vi "SATPdll.vi"(8 "error in (no error)":errorcluster, 11 "SAT Inputs":cluster{"p":dbl, "z":dbl[], "kph":u16}={"p"=0.0, "z"=[0.0, 0.0, 0.0, 0.0, 0.0, 0.0, 0.0, 0.0, 0.0, 0.0, 0.0, 0.0, 0.0, 0.0, 0.0, 0.0, 0.0, 0.0, 0.0, 0.0], "kph"=4} {"kph" items=["1 = input x is liquid composition"=1, "2 = input x is vapor composition"=2, "3 = input x is liquid composition (freezing point)"=3, "4 = input x is vapor composition (sublimation point)"=4]}) -> (0 "error out":errorcluster, 3 "SAT Outputs":T1={"D"=nan, "e"=nan, "h"=nan, "p"=nan, "s"=nan, "t"=nan, "q"=nan, "Dl"=nan, "Dv"=nan, "x"=[nan, nan, 0.0, 0.0, 0.0, 0.0, 0.0, 0.0, 0.0, 0.0, 0.0, 0.0, 0.0, 0.0, 0.0, 0.0, 0.0, 0.0, 0.0, 0.0], "y"=[nan, nan, 0.0, 0.0, 0.0, 0.0, 0.0, 0.0, 0.0, 0.0, 0.0, 0.0, 0.0, 0.0, 0.0, 0.0, 0.0, 0.0, 0.0, 0.0], "nroot"=0, "k1"=0, "t1"=nan, "p1"=nan, "d1"=nan, "k2"=0, "t2"=nan, "p2"=nan, "d2"=nan, "k3"=0, "t3"=nan, "p3"=nan, "d3"=nan, "ierr"=0, "herr"="", "herr_length"=0})   [LabVIEW 2016]
doc: "subroutine SATPdll(p, z, kph, t, dl, dv, x, y, ierr, herr, herr_length)\n\nIterate for saturated liquid and vapor states given pressure and the composition of one phase\n\nINPUTS:\n p--pressure [kPa] If T is negative, all other variables are used as initial guesses\n z--composition [array of mol frac] (phase specified by kph)\n kph--phase flag: \n 1 = input x is liquid composition (bubble point)\n 2 = input x is vapor composition (dew point)\n 3 = input x is liquid composition (freezing point)\n 4 = input x is vapor composition (sublimation point)\n\nOUTPUTS:\n t--temperature [K]\n Dl--molar density [mol/L] of saturated liquid\n Dv--molar density [mol/L] of saturated vapor\n For a pseudo pure fluid, the density of the equilibrium phase\n is not returned. Call SATP twice, once with kph=1 to get\n tliq and Dl, and once with kph=2 to get tvap and Dv.\n x--liquid phase composition [array of mol frac]\n y--vapor phase composition [array of mol frac]\n ierr--error flag: \n 0 = successful\n 2 = P < Ptp\n 4 = P < 0\n 8 = x out of range\n 12 = P and x out of range\n 140 = CRITP did not converge\n 141 = P > Pcrit\n 142 = TPRHO-liquid did not converge (pure fluid)\n 143 = TPRHO-vapor did not converge (pure fluid)\n 144 = pure fluid iteration did not converge\n The following 3 error codes are advisory--iteration will either\n converge on later guess or error out (ierr = 148)\n -144 = Raoult's law (mixture initial guess) did not converge\n -145 = TPRHO did not converge for parent ph (mix)\n -146 = TPRHO did not converge for incipient (mix)\n -147 = composition iteration did not converge\n 148 = mixture iteration did not converge\n herr--error string if ierr<>0 (character*255)\n herr_length-- length of variable herr (default: 255)"
uses:
  Ctl/SAT_Outputs.ctl
  REFPROP.DLL
panel:
  # "REFPROP-SATP_dll.vi"
  # "subroutine SATPdll(p, z, kph, t, dl, dv, x, y, ierr, herr, herr_length)"
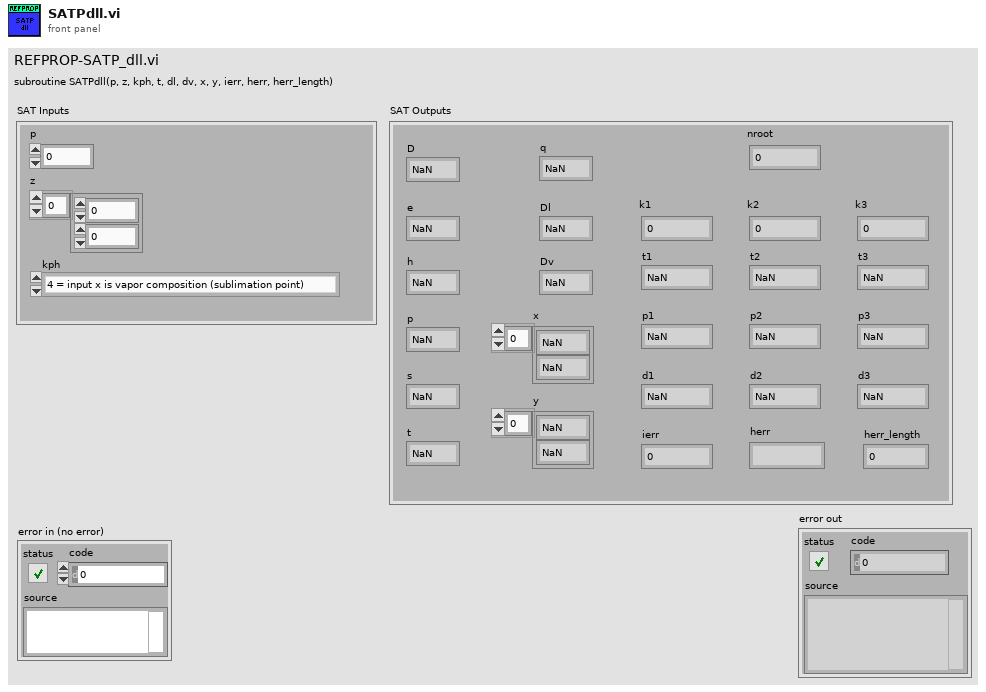
[diagram p1: front panel]
types:
  T1 = typedef "SAT_Outputs.ctl" = cluster{"D":dbl, "e":dbl, "h":dbl, "p":dbl, "s":dbl, "t":dbl, "q":dbl, "Dl":dbl, "Dv":dbl, "x":dbl[], "y":dbl[], "nroot":i32, "k1":i32, "t1":dbl, "p1":dbl, "d1":dbl, "k2":i32, "t2":dbl, "p2":dbl, "d2":dbl, "k3":i32, "t3":dbl, "p3":dbl, "d3":dbl, "ierr":i32, "herr":string, "herr_length":i32}
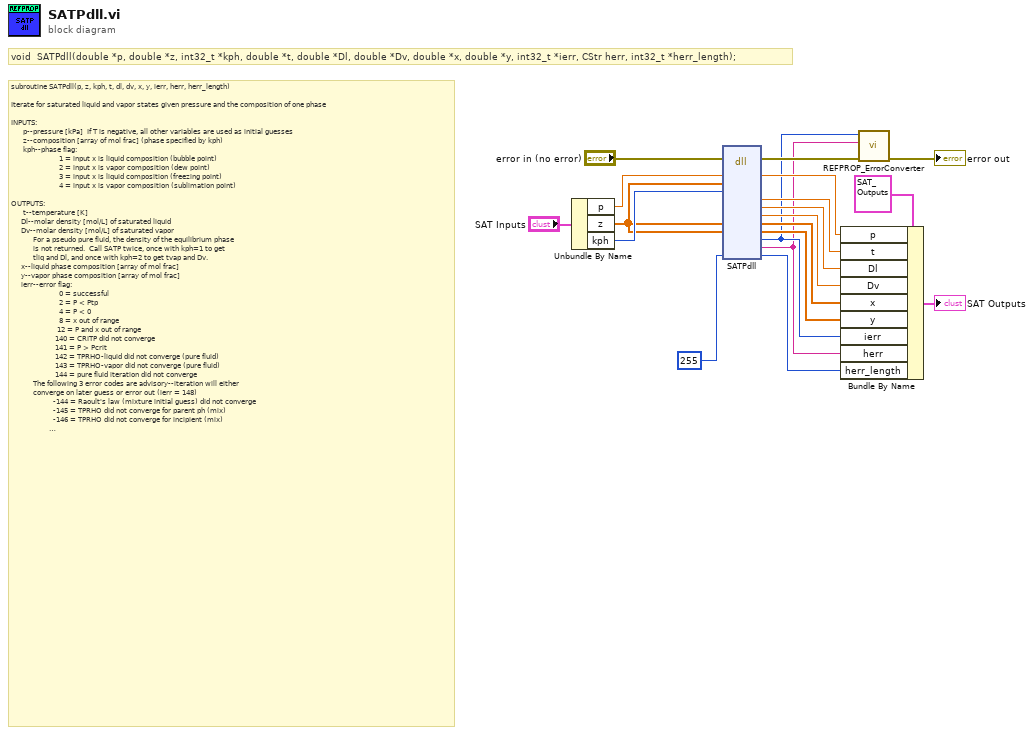
[diagram p0: block diagram]
diagram:
  # "void  SATPdll(double *p, double *z, int32_t *kph, double *t, double *Dl, double *Dv, double *x, double *y, int32_t *ierr, CStr herr, int32_t *herr_length);"
  # "subroutine SATPdll(p, z, kph, t, dl, dv, x, y, ierr, herr, herr_length)\n\nIterate for saturated liquid and vapor states given pressure and the composition of one phase\n\nINPUTS:\n      p--pressure [kPa]  If T is negative, all other variables are used as initial guesses\n      z--composition [array of mol frac] (phase specified by kph)\n      kph--phase flag:  \n                        1 = input x is liquid composition (bubble point)\n                        2 = input x is vapor composition (dew point)\n                        3 = input x is liquid composition (freezing point)\n                        4 = input x is vapor composition (sublimation point)\n\nOUTPUTS:\n      t--temperature [K]\n     Dl--molar density [mol/L] of saturated liquid\n     Dv--molar density [mol/L] of saturated vapor\n           For a pseudo pure fluid, the density of the equilibrium phase\n           is not returned.  Call SATP twice, once with kph=1 to get\n           tliq and Dl, and once with kph=2 to get tvap and Dv.\n     x--liquid phase composition [array of mol frac]\n     y--vapor phase composition [array of mol frac]\n     ierr--error flag:  \n                        0 = successful\n                        2 = P < Ptp\n                        4 = P < 0\n                        8 = x out of range\n                       12 = P and x out of range\n                      140 = CRITP did not converge\n                      141 = P > Pcrit\n                      142 = TPRHO-liquid did not converge (pure fluid)\n                      143 = TPRHO-vapor did not converge (pure fluid)\n                      144 = pure fluid iteration did not converge\n           The following 3 error codes are advisory--iteration will either\n           converge on later guess or error out (ierr = 148)\n                     -144 = Raoult's law (mixture initial guess) did not converge\n                     -145 = TPRHO did not converge for parent ph (mix)\n                     -146 = TPRHO did not converge for incipient (mix)\n                     -147 = composition iteration did not converge\n                      148 = mixture iteration did not converge\n     herr--error string if ierr<>0 (character*255)\n     herr_length-- length of variable herr (default: 255)"
  n1 = Unbundle By Name("SAT Inputs") -> ("p"=w18:dbl, "z"=w14:dbl[], "kph"=w17:u16)
  n2 = dll-call lib="C:/Program Files (x86)/REFPROP/refprop.*" fn="SATPdll"(error in="error in (no error)", "p"=w18, "z"=w14, "kph"=w17, "x"=w14, "y"=w14, "herr_length"=255 ("ln")) -> (error out=w19:errorcluster, "p"=w10:dbl, "t"=w9:dbl, "Dl"=w8:dbl, "Dv"=w7:dbl, "x"=w6:dbl[], "y"=w5:dbl[], "ierr"=w4:i32, "herr"=w3:string, "herr_length"=w2:i32)  [unwired: 10 in, 1 out]
  n3 = Bundle By Name(cluster=T1 {"D"=nan, "e"=nan, "h"=nan, "p"=nan, "s"=nan, "t"=nan, "q"=0.0, "Dl"=nan, "Dv"=nan, "x"=[nan, nan, 0.0, 0.0, 0.0, 0.0, 0.0, 0.0, 0.0, 0.0, 0.0, 0.0, 0.0, 0.0, 0.0, 0.0, 0.0, 0.0, 0.0, 0.0], "y"=[nan, nan, 0.0, 0.0, 0.0, 0.0, 0.0, 0.0, 0.0, 0.0, 0.0, 0.0, 0.0, 0.0, 0.0, 0.0, 0.0, 0.0, 0.0, 0.0], "nroot"=0, "k1"=0, "t1"=nan, "p1"=nan, "d1"=nan, "k2"=0, "t2"=nan, "p2"=nan, "d2"=nan, "k3"=0, "t3"=nan, "p3"=nan, "d3"=nan, "ierr"=0, "herr"="", "herr_length"=0} ("SAT Outputs"), "p"=w10, "t"=w9, "Dl"=w8, "Dv"=w7, "x"=w6, "y"=w5, "ierr"=w4, "herr"=w3, "herr_length"=w2) -> (→"SAT Outputs":T1)
  n4 = call "REFPROP_ErrorConverter.vi"("error in (no error)"=w19, "Error Message"=w3, "Error Code"=w4) -> ("error out"=→"error out":errorcluster)  [unwired: 8 in]
